vi "Configure Motor Speed.vi"(8 "error in (no error)":errorcluster, 10 "Motor Speed (99 : 600 RPM)":u32(ring)=99 items=["600"=99, "594"=1, "582"=2, "576"=3, "570"=4, "564"=5, "558"=6, "552"=7, "546"=8, "540"=9], 11 "VISA resource name":refnum<visa-resource-name>) -> (0 "error out":errorcluster, 3 "VISA resource name out":refnum<visa-resource-name>)   [LabVIEW 2011, in "Hokuyo URG Series.lvlib"]
doc: "The VI adjusts the motor speed in the range of 540-600 RPM in fixed increments. The default motor speed is 600 RPM. This VI is primarily used when multiple sensors are being used in the same environment to avoid light interference.\n\nNote: This VI is not supported by all devices, and an error may be returned if used on a non supported instrument."
uses:
  Hokuyo URG Series.lvlib
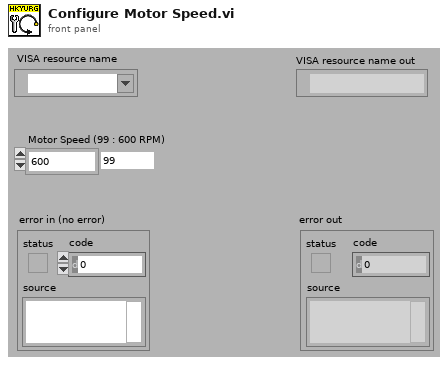
[diagram p1: front panel]
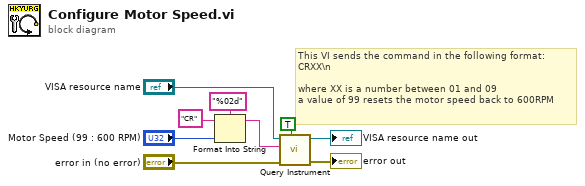
[diagram p0: block diagram]
diagram:
  # "This VI sends the command in the following format:\nCRXX\\n\n\nwhere XX is a number between 01 and 09\na value of 99 resets the motor speed back to 600RPM"
  n1 = Format Into String(format string="%02d", initial string="CR", "Motor Speed (99 : 600 RPM)") -> (resulting string=w8:string)  [unwired: 1 in, 1 out]
  n2 = call "Query Instrument.vi"("Error Query (Enabled)"=TRUE, "error in"="error in (no error)", "Command"=w8, "VISA Resource Name"="VISA resource name") -> ("error out"=→"error out":errorcluster, "VISA Resource Name Out"=→"VISA resource name out":refnum<visa-resource-name>)  [unwired: 5 in, 1 out]
